vi "time_stamp.vi"(11 "入力ピン":bool) -> (3 "出力値":T1)   [LabVIEW 2023]
uses:
  <vilib>/Utility/miscctls.llb/LVDateTimeRec.ctl
panel:
  in  "Button SW":bool
  out "出力値":T1
  in  "曜日表示設定":enum32{"なし", "（月）", "（Mon）", "月曜日"}(tab)
  out "曜日なしの場合の表示":string
  out "（曜日）表示":string
  out "（英語略）表示":string
  out "漢字表示":string
  in  "時間表示設定":T2(tab)
  out "時間と分を表示":string
  out "時間と分と秒を表示":string
  out "時間と分と秒を表示※秒は1/1000秒（ｍS）まで表示":string
  out "時間と分と秒を表示※秒は最小分解能（uS）で表示":string
  out "Get Date/Time Stringパレットを使った時間と分の表示":string
  out "タイムスタンプ値":T3
  # "１秒以下の値"
  # "秒"
  # "分"
  # "時"
  # "日"
  # "月"
  # "年"
  # "曜日表、時間表示の設定は表示したいタブを選択して保存することで設定したことになります。"
  # "曜日を数値化"
  # "今年の１月１日から数えた日数"
  # "サマータイムについての値\n※日本は現在サマータイムがないので０"
  # "."
  # "."
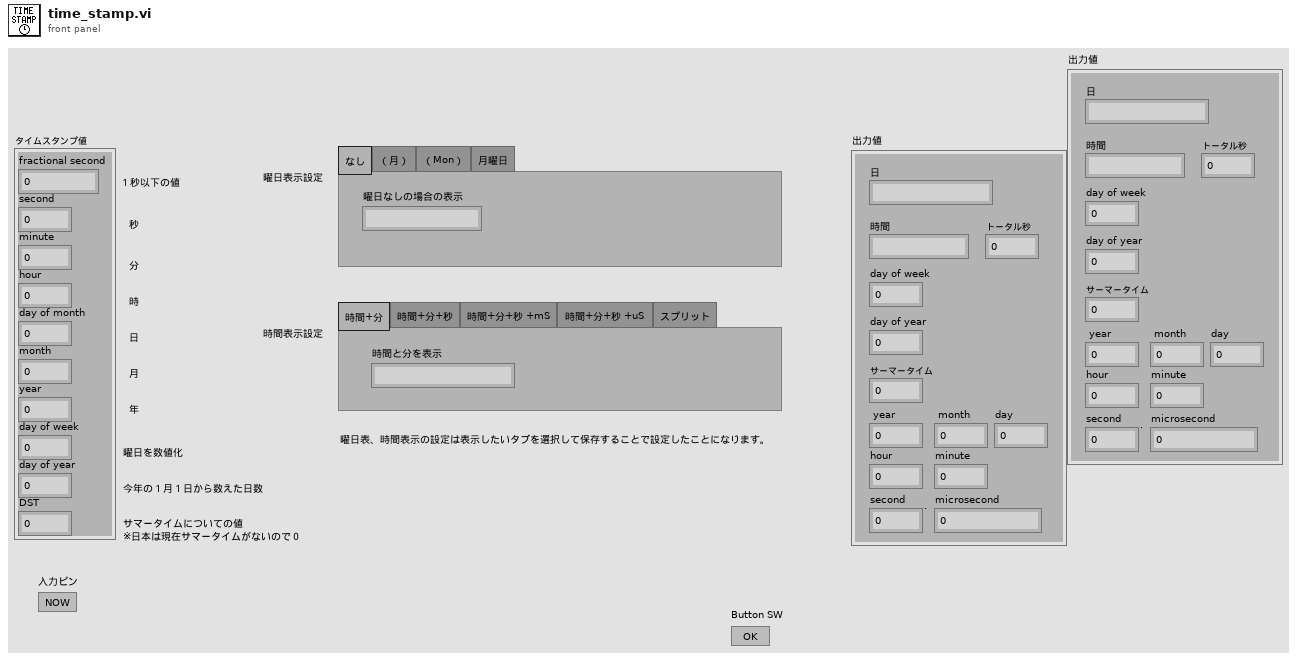
[diagram p1: front panel]
types:
  T1 = cluster{"日":string, "トータル秒":i32, "時間":string, "day of week":i32, "day of year":i32, "サーマータイム":i32, "hour":i32, "minute":i32, "second":i32, "day":i32, " month":i32, " year":i32, "microsecond":i32}
  T2 = enum32{"時間+分", "時間+分+秒", "時間+分+秒 +mS", "時間+分+秒 +uS ", "スプリット"}
  T3 = typedef "LVDateTimeRec.ctl" = cluster{"fractional second":dbl, "second":i32, "minute":i32, "hour":i32, "day of month":i32, "month":i32, "year":i32, "day of week":i32, "day of year":i32, "DST":i32}
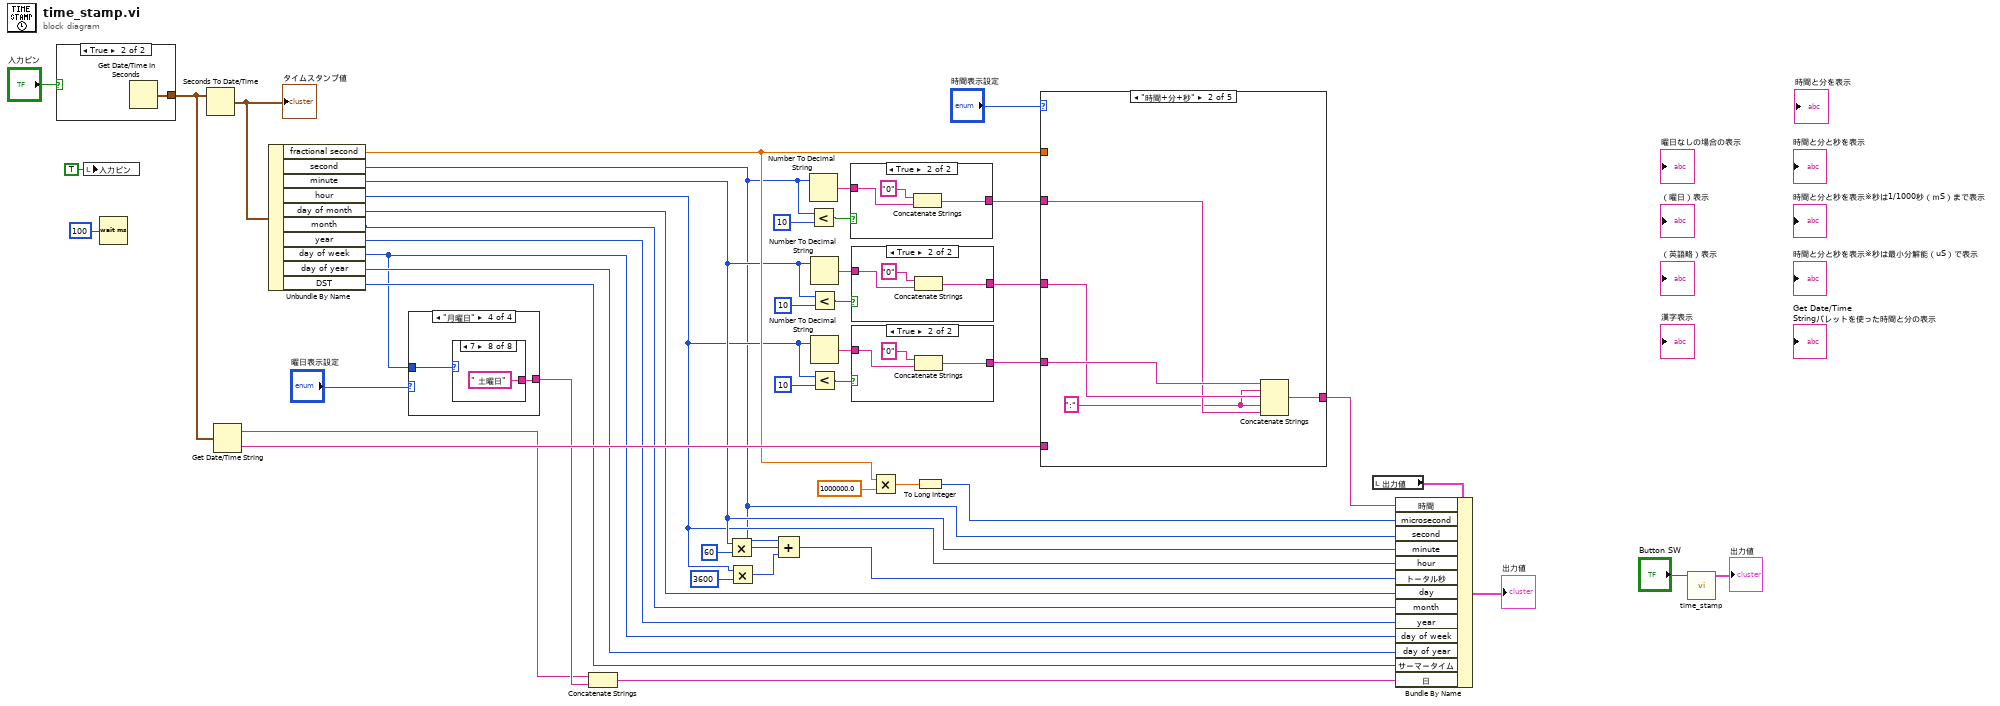
[diagram p0: block diagram]
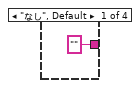
[diagram p2: hidden frame]
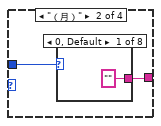
[diagram p3: hidden frame]
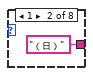
[diagram p4: hidden frame]
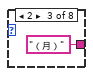
[diagram p5: hidden frame]
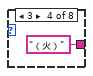
[diagram p6: hidden frame]
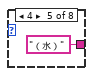
[diagram p7: hidden frame]
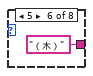
[diagram p8: hidden frame]
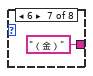
[diagram p9: hidden frame]
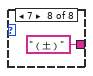
[diagram p10: hidden frame]
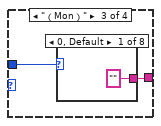
[diagram p11: hidden frame]
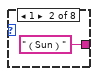
[diagram p12: hidden frame]
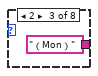
[diagram p13: hidden frame]
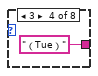
[diagram p14: hidden frame]
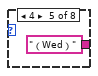
[diagram p15: hidden frame]
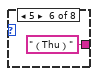
[diagram p16: hidden frame]
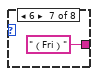
[diagram p17: hidden frame]
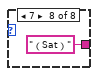
[diagram p18: hidden frame]
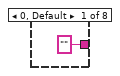
[diagram p19: hidden frame]
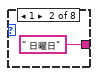
[diagram p20: hidden frame]
diagram:
  n1 = case shown="True" "入力ピン" {
    tunnel: [timestamp(0 s since 1904-01-01) w48] -> w29
    frame False {
    }
    frame True {
      n2 = Get Date/Time In Seconds() -> (seconds since 1Jan1904=w48:timestamp)
    }
  }
  n3 = local write "入力ピン"(TRUE ("Button")) -> ()
  n4 = Wait (ms)(milliseconds to wait=u32 100) -> ()  [unwired: 1 out]
  n5 = Seconds To Date/Time(time stamp (now)=w29) -> (date time rec=w25:T3)  [unwired: 1 in]
  "タイムスタンプ値" <- w25
  n6 = Get Date/Time String(seconds (now)=w29) -> (date string=w22:string, time string=w42:string)  [unwired: 2 in]
  n7 = Unbundle By Name(w25) -> ("fractional second"=w17:dbl, "second"=w3:i32, "minute"=w15:i32, "hour"=w14:i32, "day of month"=w12:i32, "month"=w7:i32, "year"=w6:i32, "day of week"=w8:i32, "day of year"=w9:i32, "DST"=w10:i32)
  n8 = case shown="\"月曜日\"" "曜日表示設定" {
    tunnel: ["" w50 w60 w70] -> w23
    tunnel: w8 -> [_ w51 w61 w71]
    frame "なし", Default {
    }
    frame "（月）" {
      n9 = case shown="0, Default" w51 {
        tunnel: ["" "（日）" "（月）" "（火）" "（水）" "（木）" "（金）" "（土）"] -> w50
        frame 0, Default {
        }
        frame 1 {
        }
        frame 2 {
        }
        frame 3 {
        }
        frame 4 {
        }
        frame 5 {
        }
        frame 6 {
        }
        frame 7 {
        }
      }
    }
    frame "（Mon）" {
      n10 = case shown="0, Default" w61 {
        tunnel: ["" "（Sun）" "（Mon）" "（Tue）" "（Wed）" "（Thu）" "（Fri）" "（Sat）"] -> w60
        frame 0, Default {
        }
        frame 1 {
        }
        frame 2 {
        }
        frame 3 {
        }
        frame 4 {
        }
        frame 5 {
        }
        frame 6 {
        }
        frame 7 {
        }
      }
    }
    frame "月曜日" {
      n11 = case shown="7" w71 {
        tunnel: ["" " 日曜日" " 月曜日" " 火曜日" " 水曜日" " 木曜日" " 金曜日" " 土曜日"] -> w70
        frame 0, Default {
        }
        frame 1 {
        }
        frame 2 {
        }
        frame 3 {
        }
        frame 4 {
        }
        frame 5 {
        }
        frame 6 {
        }
        frame 7 {
        }
      }
    }
  }
  n12 = Concatenate Strings(w22, w23) -> (w11:string)
  n13 = Multiply(x=w15, y=60) -> (x*y=w44:i32)
  n14 = Multiply(x=w14, y=3600) -> (x*y=w43:i32)
  n15 = Compound Arithmetic op=ADD(w3, w44, w43) -> (w13:i32)
  n16 = Number To Decimal String(number=w3) -> (decimal integer string=w40:string)  [unwired: 1 in]
  n17 = Less?(x=w3, y=10) -> (x < y?=w41:bool)
  n18 = Number To Decimal String(number=w15) -> (decimal integer string=w36:string)  [unwired: 1 in]
  n19 = Less?(x=w15, y=10) -> (x < y?=w37:bool)
  n20 = Number To Decimal String(number=w14) -> (decimal integer string=w33:string)  [unwired: 1 in]
  n21 = Less?(x=w14, y=10) -> (x < y?=w34:bool)
  n22 = case shown="True" w41 {
    tunnel: w40 -> [w80 w83]
    tunnel: [w80 w82] -> w38
    frame False {
    }
    frame True {
      n23 = Concatenate Strings("0" ("string"), w83) -> (w82:string)
    }
  }
  n24 = case shown="True" w37 {
    tunnel: w36 -> [w84 w87]
    tunnel: [w84 w86] -> w30
    frame False {
    }
    frame True {
      n25 = Concatenate Strings("0" ("string"), w87) -> (w86:string)
    }
  }
  n26 = case shown="True" w34 {
    tunnel: w33 -> [w88 w91]
    tunnel: [w88 w90] -> w31
    frame False {
    }
    frame True {
      n27 = Concatenate Strings("0" ("string"), w91) -> (w90:string)
    }
  }
  n28 = Multiply(x=w17, y=1000000.0) -> (x*y=w16:dbl)
  n29 = To Long Integer(number=w16) -> (32bit integer=w4:i32)
  n30 = case shown="\"時間+分+秒\"" "時間表示設定" {
    tunnel: w38 -> [_ w97 w110 w120 _]
    tunnel: w30 -> [w93 w99 w111 w121 _]
    tunnel: w31 -> [w92 w100 w112 w122 _]
    tunnel: [w94 w98 w108 w118 w124] -> w5
    tunnel: w17 -> [_ _ w104 w114 _]
    tunnel: w42 -> [_ _ _ _ w124]
    frame "時間+分", Default {
      n31 = Concatenate Strings(w92, ":" ("string"), w93) -> (w94:string)
    }
    frame "時間+分+秒" {
      w96 = ":" ("string")
      n32 = Concatenate Strings(w100, w96, w99, w96, w97) -> (w98:string)
    }
    frame "時間+分+秒 +mS" {
      w109 = ":" ("string")
      n33 = Multiply(x=w104, y=1000.0) -> (x*y=w107:dbl)
      n34 = Round To Nearest(number=w107) -> (nearest integer value=w105:dbl)
      n35 = To Long Integer(number=w105) -> (32bit integer=w101:i32)
      n36 = Number To Decimal String(number=w101) -> (decimal integer string=w102:string)  [unwired: 1 in]
      n37 = Concatenate Strings(w112, w109, w111, w109, w110, "." ("string"), w102) -> (w108:string)
    }
    frame "時間+分+秒 +uS " {
      w123 = ":" ("string")
      n38 = Multiply(x=w114, y=1000000.0) -> (x*y=w115:dbl)
      n39 = To Long Integer(number=w115) -> (32bit integer=w116:i32)
      n40 = Number To Decimal String(number=w116) -> (decimal integer string=w117:string)  [unwired: 1 in]
      n41 = Concatenate Strings(w122, w123, w121, w123, w120, "." ("string"), w117) -> (w118:string)
    }
    frame "スプリット" {
    }
  }
  n42 = local read "出力値"() -> (w20:T1)
  n43 = Bundle By Name(cluster=w20, "時間"=w5, "microsecond"=w4, "second"=w3, "minute"=w15, "hour"=w14, "トータル秒"=w13, "day"=w12, "month"=w7, "year"=w6, "day of week"=w8, "day of year"=w9, "サーマータイム"=w10, "日"=w11) -> (→"出力値":T1)
  n44 = call "time_stamp.vi"("入力ピン"="Button SW") -> ("出力値"=→"出力値":T1)  [unwired: 10 in]
